vi "DragDropMoveCopy.vi"(0 "Type":T1=enum."Value Change", 1 "Allowed Parent Child":set{cluster{"Parent":i32, "Child":i32}}(c389), 2 "Bar Cursor ID":refnum<k1>, 3 "Max Column Count (10)":i32=10, 5 "Drag Status":T3, 7 "CtlRef":refnum<vi>, 9 "InBounds in":bool, 11 "error in":errorcluster, 12 "PlatMods":T2, 13 "Available Data Names":string[](array[string])) -> (4 "CtlRef out":refnum<vi>, 6 "Data Tag":string, 8 "Parent Tag":string, 10 "Insert Index":i32, 14 "Accepted?":bool, 15 "error out":errorcluster)   [LabVIEW 2019, in "TreeControlLib.lvlib"]
uses:
  TreeControlLib.lvlib
  79e01bdc-b2b9-467f-8444-051767dc36a0.vi
  <vilib>/Utility/cursorutil.llb/Set Cursor (Icon Pict).vi
  <vilib>/Utility/cursorutil.llb/Set Cursor (Cursor ID).vi
  <vilib>/event_ctls.llb/lveventtype.ctl
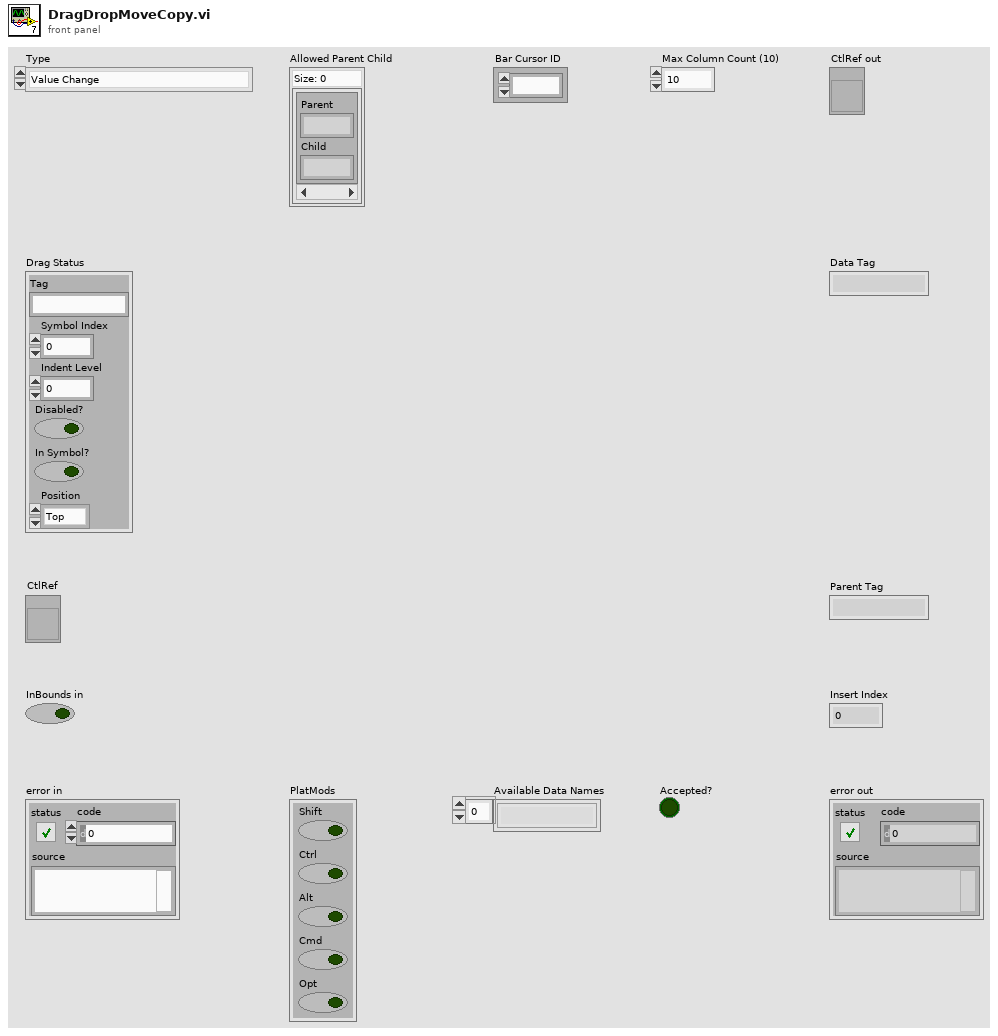
[diagram p1: front panel]
types:
  T1 = typedef "lveventtype.ctl" = enum32{"Null", "Timeout", "Annotation Menu Selection", "Annotation Menu Selection?", "App Instance Close", "App Instance Close?", "Autoscale Range Change", "Bookmark Info Change", "Cell Edit", "Cell Edit?", "Cursor Grab", "Cursor Grab?", "Cursor Menu Selection", "Cursor Menu Selection?", "Cursor Move", "Cursor Release", "Data Change", "Direction Change", "Display State Change", "Drag Ended", "Drag Enter", "Drag Leave", "Drag Over", "Drag Source Update", "Drag Starting", "Drag Starting?", "Drop", "Exec State Change", "Key Down", "Key Down?", "Key Repeat", "Key Repeat?", "Key Up", "Listbox Double Click", "Menu Activation?", "Menu Selection (App)", "Menu Selection? (App)", "Menu Selection (User)", "Mouse Down", "Mouse Down?", "Mouse Enter", "Mouse Leave", "Mouse Move", "Mouse Up", "Mouse Wheel", "NI Security User Change (App)", "Pane Size", "Panel Close", "Panel Close?", "Panel Resize", "Plot Attribute Change", "Scale Range Change", "Shortcut Menu Activation?", "Shortcut Menu Selection (App)", "Shortcut Menu Selection? (App)", "Shortcut Menu Selection (User)", "Tree Double Click", "Tree Drag", "Tree Drag?", "Tree Drop", "Tree Drop?", "Tree Item Close", "Tree Item Close?", "Tree Item Open", "Tree Item Open?", "User Event", "Value Change"}
  T2 = cluster{"Shift":bool, "Ctrl":bool, "Alt":bool, "Cmd":bool, "Opt":bool}
  T3 = cluster{"Tag":string, "Symbol Index":i32, "Indent Level":i32, "Disabled?":bool, "In Symbol?":bool, "Position":enum16{"Top", "Center", "Bottom"}}
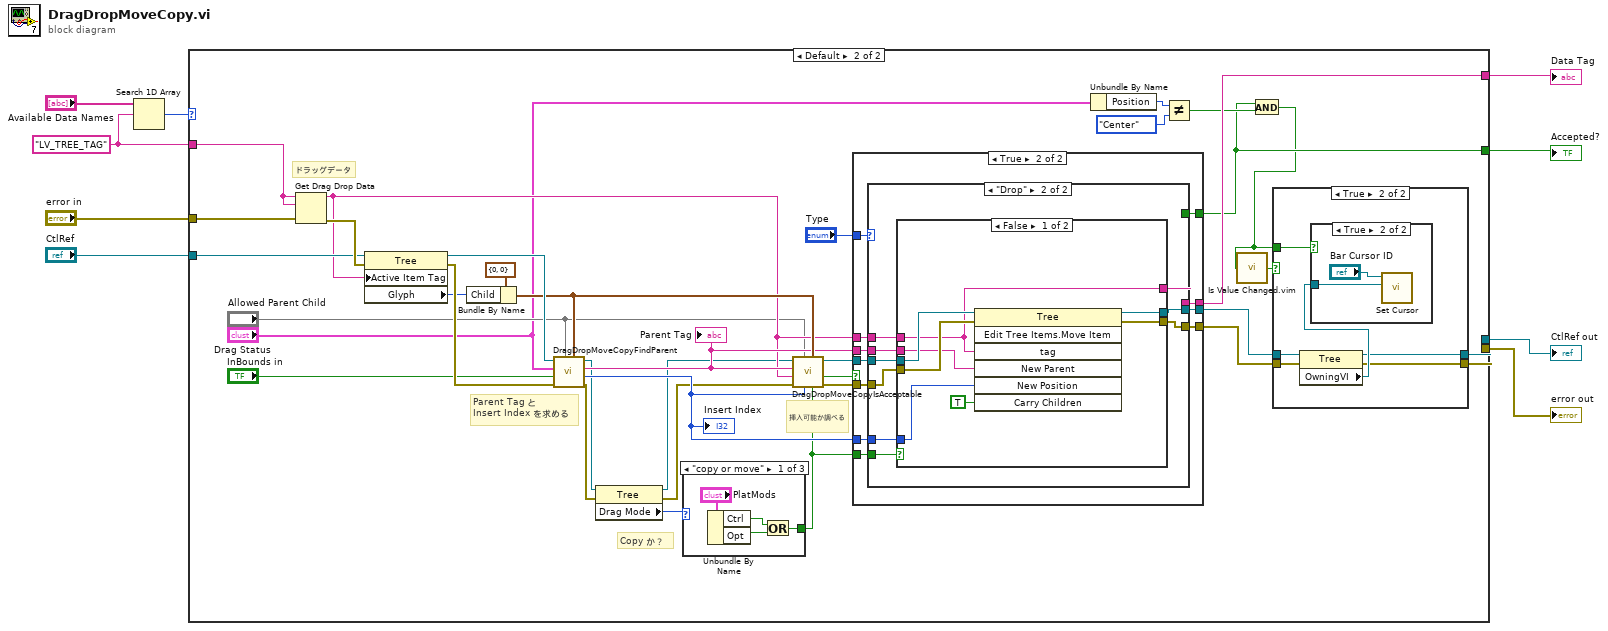
[diagram p0: block diagram]
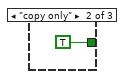
[diagram p3: hidden frame]
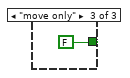
[diagram p4: hidden frame]
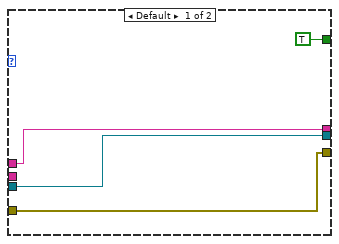
[diagram p6: hidden frame]
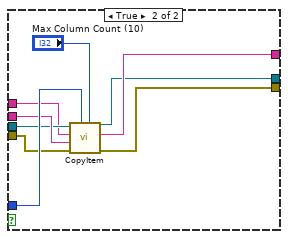
[diagram p7: hidden frame]
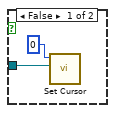
[diagram p9: hidden frame]
diagram:
  w8 = "LV_TREE_TAG"
  n1 = Search 1D Array(1D array="Available Data Names", element=w8) -> (index of element=w7:i32)  [unwired: 1 in]
  n2 = case shown="Default" w7 {
    tunnel: w8 -> [_ w41]
    tunnel: "error in" -> [w10 w40]
    tunnel: "CtlRef" -> [w11 w39]
    tunnel: [_ w31] -> w4
    tunnel: [w11 w26] -> w3
    tunnel: [w10 w25] -> w2
    tunnel: [_ w21] -> w1
    frame -1 {
    }
    frame Default {
      # "Copy か？"
      # "挿入可能か調べる"
      # "Parent Tag と\nInsert Index を求める"
      # "ドラッグデータ"
      n3 = Get Drag Drop Data(6:w40, 8:w41, 9:w41) -> (0:w47:errorcluster, 3:w32:string)
      n4 = property class="Tree"(reference=w39, error in=w47, "Active Item Tag"=w32) -> (reference out=w38:refnum<vi>, error out=w46:errorcluster, "Glyph"=w45:i32)
      n5 = Bundle By Name(cluster=cluster{"Parent":i32, "Child":i32} {"Parent"=0, "Child"=0} ("element"), "Child"=w45) -> (w36:cluster{"Parent":i32, "Child":i32})
      n6 = call "DragDropMoveCopyFindParent.vi"("ParentChild"=w36, "Allowed Parent Child"="Allowed Parent Child", "error in (no error)"=w46, "InBounds"="InBounds in", "Drag Status"="Drag Status", "TreeControl in"=w38) -> ("error out"=w13:errorcluster, "Insert Inex"=w18:i32, "Parent Tag"=w33:string, "TreeControl out"=w16:refnum<vi>)  [unwired: 2 in]
      "Parent Tag" <- w33
      "Insert Index" <- w18
      n7 = property class="Tree"(reference=w16, error in=w13) -> (reference out=w15:refnum<vi>, error out=w12:errorcluster, "Drag Mode"=w17:enum32{"copy or move", "copy only", "move only"})
      n8 = case shown="\"copy or move\"" w17 {
        tunnel: [w48 TRUE FALSE] -> w14
        frame "copy or move" {
          n9 = Unbundle By Name("PlatMods") -> ("Ctrl"=w50:bool, "Opt"=w51:bool)
          n10 = Or(x=w50, y=w51) -> (x .or. y?=w48:bool)
        }
        frame "copy only" {
        }
        frame "move only" {
        }
      }
      n11 = call "DragDropMoveCopyIsAcceptable.vi"("Copy?"=w14, "element"=w36, "Insert Index"=w18, "Allowed Parent Child"="Allowed Parent Child", "error in (no error)"=w12, "Data Tag"=w32, "Parent Tag"=w33, "TreeControl in"=w15) -> ("error out"=w42:errorcluster, "Acceptable"=w35:bool, "TreeControl out"=w43:refnum<vi>)  [unwired: 1 in]
      n12 = case shown="True" w35 {
        tunnel: w43 -> [w55 w67]
        tunnel: w42 -> [w54 w66]
        tunnel: "Type" -> [_ w65]
        tunnel: w33 -> [_ w64]
        tunnel: w32 -> [w56 w63]
        tunnel: w18 -> [_ w62]
        tunnel: [w56 w61] -> w31
        tunnel: [w55 w60] -> w29
        tunnel: [w54 w59] -> w28
        tunnel: [_ w58] -> w21
        tunnel: w14 -> [_ w57]
        frame False {
        }
        frame True {
          n13 = case shown="\"Drop\"" w65 {
            tunnel: w67 -> [w69 w72]
            tunnel: w66 -> [w68 w73]
            tunnel: w64 -> [_ w80]
            tunnel: w63 -> [w70 w79]
            tunnel: w62 -> [_ w78]
            tunnel: [w70 w77] -> w61
            tunnel: [w69 w76] -> w60
            tunnel: [w68 w75] -> w59
            tunnel: [TRUE _] -> w58
            tunnel: w57 -> [_ w74]
            frame Default {
            }
            frame "Drop" {
              n14 = case shown="False" w74 {
                tunnel: w72 -> [w88 w95]
                tunnel: w73 -> [w87 w94]
                tunnel: w80 -> [w86 w96]
                tunnel: w79 -> [w83 w93]
                tunnel: w78 -> [w85 w97]
                tunnel: [w83 w91] -> w77
                tunnel: [w82 w89] -> w75
                tunnel: [w81 w90] -> w76
                frame False {
                  n15 = invoke class="Tree" method="Edit Tree Items.Move Item"(reference=w88, error in=w87, "tag"=w83, "New Parent"=w86, "New Position"=w85, "Carry Children"=TRUE ("Carry Children?")) -> (reference out=w81:refnum<vi>, error out=w82:errorcluster)  [unwired: 1 in, 5 out]
                }
                frame True {
                  n16 = call "CopyItem.vi"("Max Column Count (10)"="Max Column Count (10)", "Insert Inex"=w97, "error in (no error)"=w94, "Parent Tag"=w96, "Source Tag"=w93, "TreeControl in"=w95) -> ("error out"=w89:errorcluster, "Copied Tag"=w91:string, "TreeControl out"=w90:refnum<vi>)  [unwired: 3 in]
                }
              }
            }
          }
        }
      }
      n17 = Unbundle By Name("Drag Status") -> ("Position"=w24:enum16{"Top", "Center", "Bottom"})
      n18 = Not Equal?(x=w24, y=enum16{"Top", "Center", "Bottom"}."Center" ("Position")) -> (x != y?=w22:bool)
      n19 = And(x=w21, y=w22) -> (x .and. y?=w19:bool)
      n20 = call "Is Value Changed.vim"("value"=w19) -> ("changed or first call?"=w27:bool)
      n21 = case shown="True" w27 {
        tunnel: w29 -> [w99 w105]
        tunnel: w28 -> [w98 w104]
        tunnel: [w99 w102] -> w26
        tunnel: [w98 w101] -> w25
        tunnel: w19 -> [_ w100]
        frame False {
        }
        frame True {
          n22 = property class="Tree"(reference=w105, error in=w104) -> (reference out=w102:refnum<vi>, error out=w101:errorcluster, "OwningVI"=w103:refnum<vi>)
          n23 = case shown="True" w100 {
            tunnel: w103 -> [w107 w109]
            frame False {
              n24 = call-poly <vilib>:"Set Cursor.vi"("VI reference (current VI)"=w107, "icon"=0) -> ()  [unwired: 8 in, 2 out]
            }
            frame True {
              n25 = call-poly <vilib>:"Set Cursor.vi"("VI reference (current VI)"=w109, "cursor ID"="Bar Cursor ID") -> ()  [unwired: 8 in, 2 out]
            }
          }
        }
      }
    }
  }
  "Accepted?" <- w1
  "error out" <- w2
  "Data Tag" <- w4
  "CtlRef out" <- w3
